vi "Report - Flow Control.vi"(0 "Log Folder Path (Create Log)":path, 1 "DUT Number":i32, 2 "Text Input":string[](array[string]), 3 "WLAN TX Result":T8, 4 "WLAN RX Result":T7, 5 "error in":errorcluster, 6 "Reprot Log Flow Control":T6, 7 "DUT log path":path, 8 "TV Parameters(DataType)":T1 {"Standard" items=["80211A/G/J/P OFDM", "80211B/G DSSS", "80211G DSSSOFDM", "80211N MIMOOFDM", "80211AC MIMOOFDM"]; "OFDM Data Rate (Mbps)" items=["6", "9", "12", "18", "24", "36", "48", "54"]; "80211n PLCP Frame Format" items=["Mixed Format", "Greenfield Format"]; "FEC Coding Type" items=["BCC", "LDPC"]; "DSSS Data Rate (Mbps)" items=["1", "2", "5.5 CCK", "5.5 PBCC", "11 CCK", "11 PBCC", "22", "33"]}) -> (14 "Pass or not":bool, 15 "Text Output":string[](array[string]), 16 "Cluster 2":T2, 17 "DUT1 log path":path, 19 "error out":errorcluster)   [LabVIEW 2014]
uses:
  TypeDef/Report Log Flow Control.ctl
  TV/RW/Includes/WLAN - TV - RW - INC - TV_DataType_Cluster.ctl
  TypeDef/DUT Number.ctl
  <vilib>/Utility/file.llb/Write To Spreadsheet File (string).vi
  <vilib>/Utility/file.llb/Read From Spreadsheet File (string).vi
panel:
  out "DUT1 Results":string[][](array[string])
  out "Text Output":string[][](array[string])
  in  "BT RX Result":T3
  in  "BT TX EDR Result":T4 {"EDR_OMEGA_I (Hz)" format="%.2g"; "EDR_PROB_EVM_99_PASS (%)" format="%.2g"; "EDR_EVM_PK (%)" format="%.2g"; "EDR_EVM_AV (%)" format="%.2g"; "EDR_POW_DIFF_DB (dB)" format="%.2f"; "POWER_PEAK_DBM (dBm)" format="%.2f"; "POWER_AVERAGE_DBM (dBm)" format="%.2f"}
  in  "BT TX BR Result":T5 {"FREQ_EST_HEADER  (Hz)" format="%^.3g"; "FREQ_EST (Hz)" format="%^.3e"; "FREQ_DRIFT (Hz)" format="%^.3e"; "DELTA_F2_MAX_ACCESS (Hz)" format="%^.3e"; "DELTA_F2_AVERAGE (Hz)" format="%^.3e"; "POWER_PEAK_DBM (dBm)" format="%.2f"; "POWER_AVERAGE_DBM (dBm)" format="%.2f"; "DELTA_F1_AVERAGE (Hz)" format="%^.3e"}
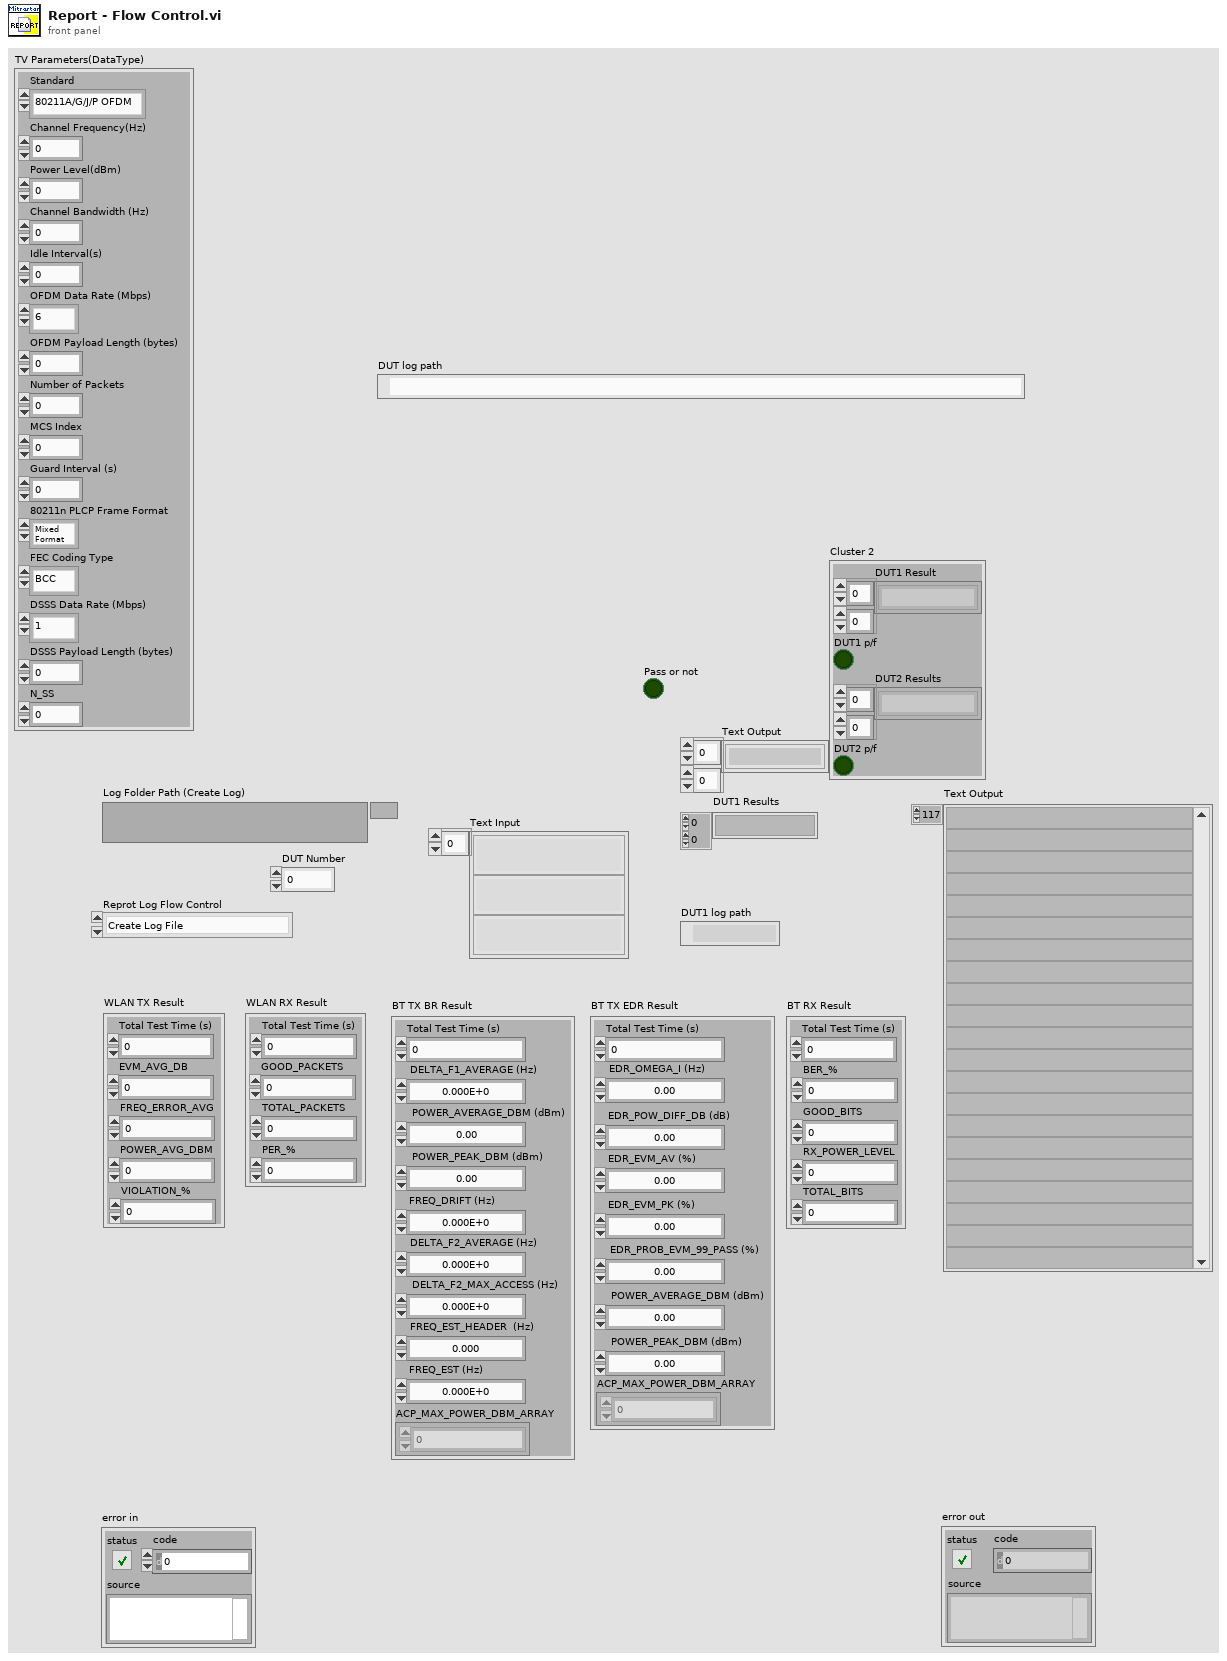
[diagram p1: front panel]
types:
  T1 = typedef "WLAN - TV - RW - INC - TV_DataType_Cluster.ctl" = cluster{"Standard":i32, "Channel Frequency(Hz)":dbl, "Power Level(dBm)":dbl, "Channel Bandwidth (Hz)":dbl, "Idle Interval(s)":dbl, "OFDM Data Rate (Mbps)":i32, "OFDM Payload Length (bytes)":i32, "Number of Packets":i32, "MCS Index":i32, "Guard Interval (s)":dbl, "80211n PLCP Frame Format":i32, "FEC Coding Type":i32, "DSSS Data Rate (Mbps)":i32, "DSSS Payload Length (bytes)":i32, "N_SS":i32}
  T2 = cluster{"DUT1 Result":string[][], "DUT1 p/f":bool, "DUT2 Results":string[][], "DUT2 p/f":bool}
  T3 = cluster{"Total Test Time (s)":dbl, "BER_%":dbl, "GOOD_BITS":i32, "RX_POWER_LEVEL":dbl, "TOTAL_BITS":i32}
  T4 = cluster{"Total Test Time (s)":dbl, "EDR_OMEGA_I (Hz)":dbl, "EDR_POW_DIFF_DB (dB)":dbl, "EDR_EVM_AV (%)":dbl, "EDR_EVM_PK (%)":dbl, "EDR_PROB_EVM_99_PASS (%)":dbl, "POWER_AVERAGE_DBM (dBm)":dbl, "POWER_PEAK_DBM (dBm)":dbl, "ACP_MAX_POWER_DBM_ARRAY":dbl[]}
  T5 = cluster{"Total Test Time (s)":dbl, "DELTA_F1_AVERAGE (Hz)":dbl, "POWER_AVERAGE_DBM (dBm)":dbl, "POWER_PEAK_DBM (dBm)":dbl, "FREQ_DRIFT (Hz)":dbl, "DELTA_F2_AVERAGE (Hz)":dbl, "DELTA_F2_MAX_ACCESS (Hz)":dbl, "FREQ_EST_HEADER  (Hz)":dbl, "FREQ_EST (Hz)":dbl, "ACP_MAX_POWER_DBM_ARRAY":dbl[]}
  T6 = typedef "Report Log Flow Control.ctl" = enum16{"Create Log File", "Append Test Item Head", "Append WLAN TX IQ Result", "Append WLAN TX Spectrum Result", "Append WLAN RX Result", "Append BT TX BR Result", "Append BT TX EDR Result", "Append Customized Text", "Append BT RX Result", "Read Log File", "Save Test Time"}
  T7 = cluster{"Total Test Time (s)":dbl, "GOOD_PACKETS":i32, "TOTAL_PACKETS":i32, "PER_%":dbl}
  T8 = cluster{"Total Test Time (s)":dbl, "EVM_AVG_DB":dbl, "FREQ_ERROR_AVG":dbl, "POWER_AVG_DBM":dbl, "VIOLATION_%":dbl}
  T9 = typedef "DUT Number.ctl" = string
  T10 = cluster{"all rows":string[][], "p/f":bool, "all rows":string[][], "p/f":bool}
  T11 = cluster{"POWER_AVG_DBM":string, "EVM_AVG_DB":string, "FREQ_ERROR_AVG":string, "RX_PER":string}
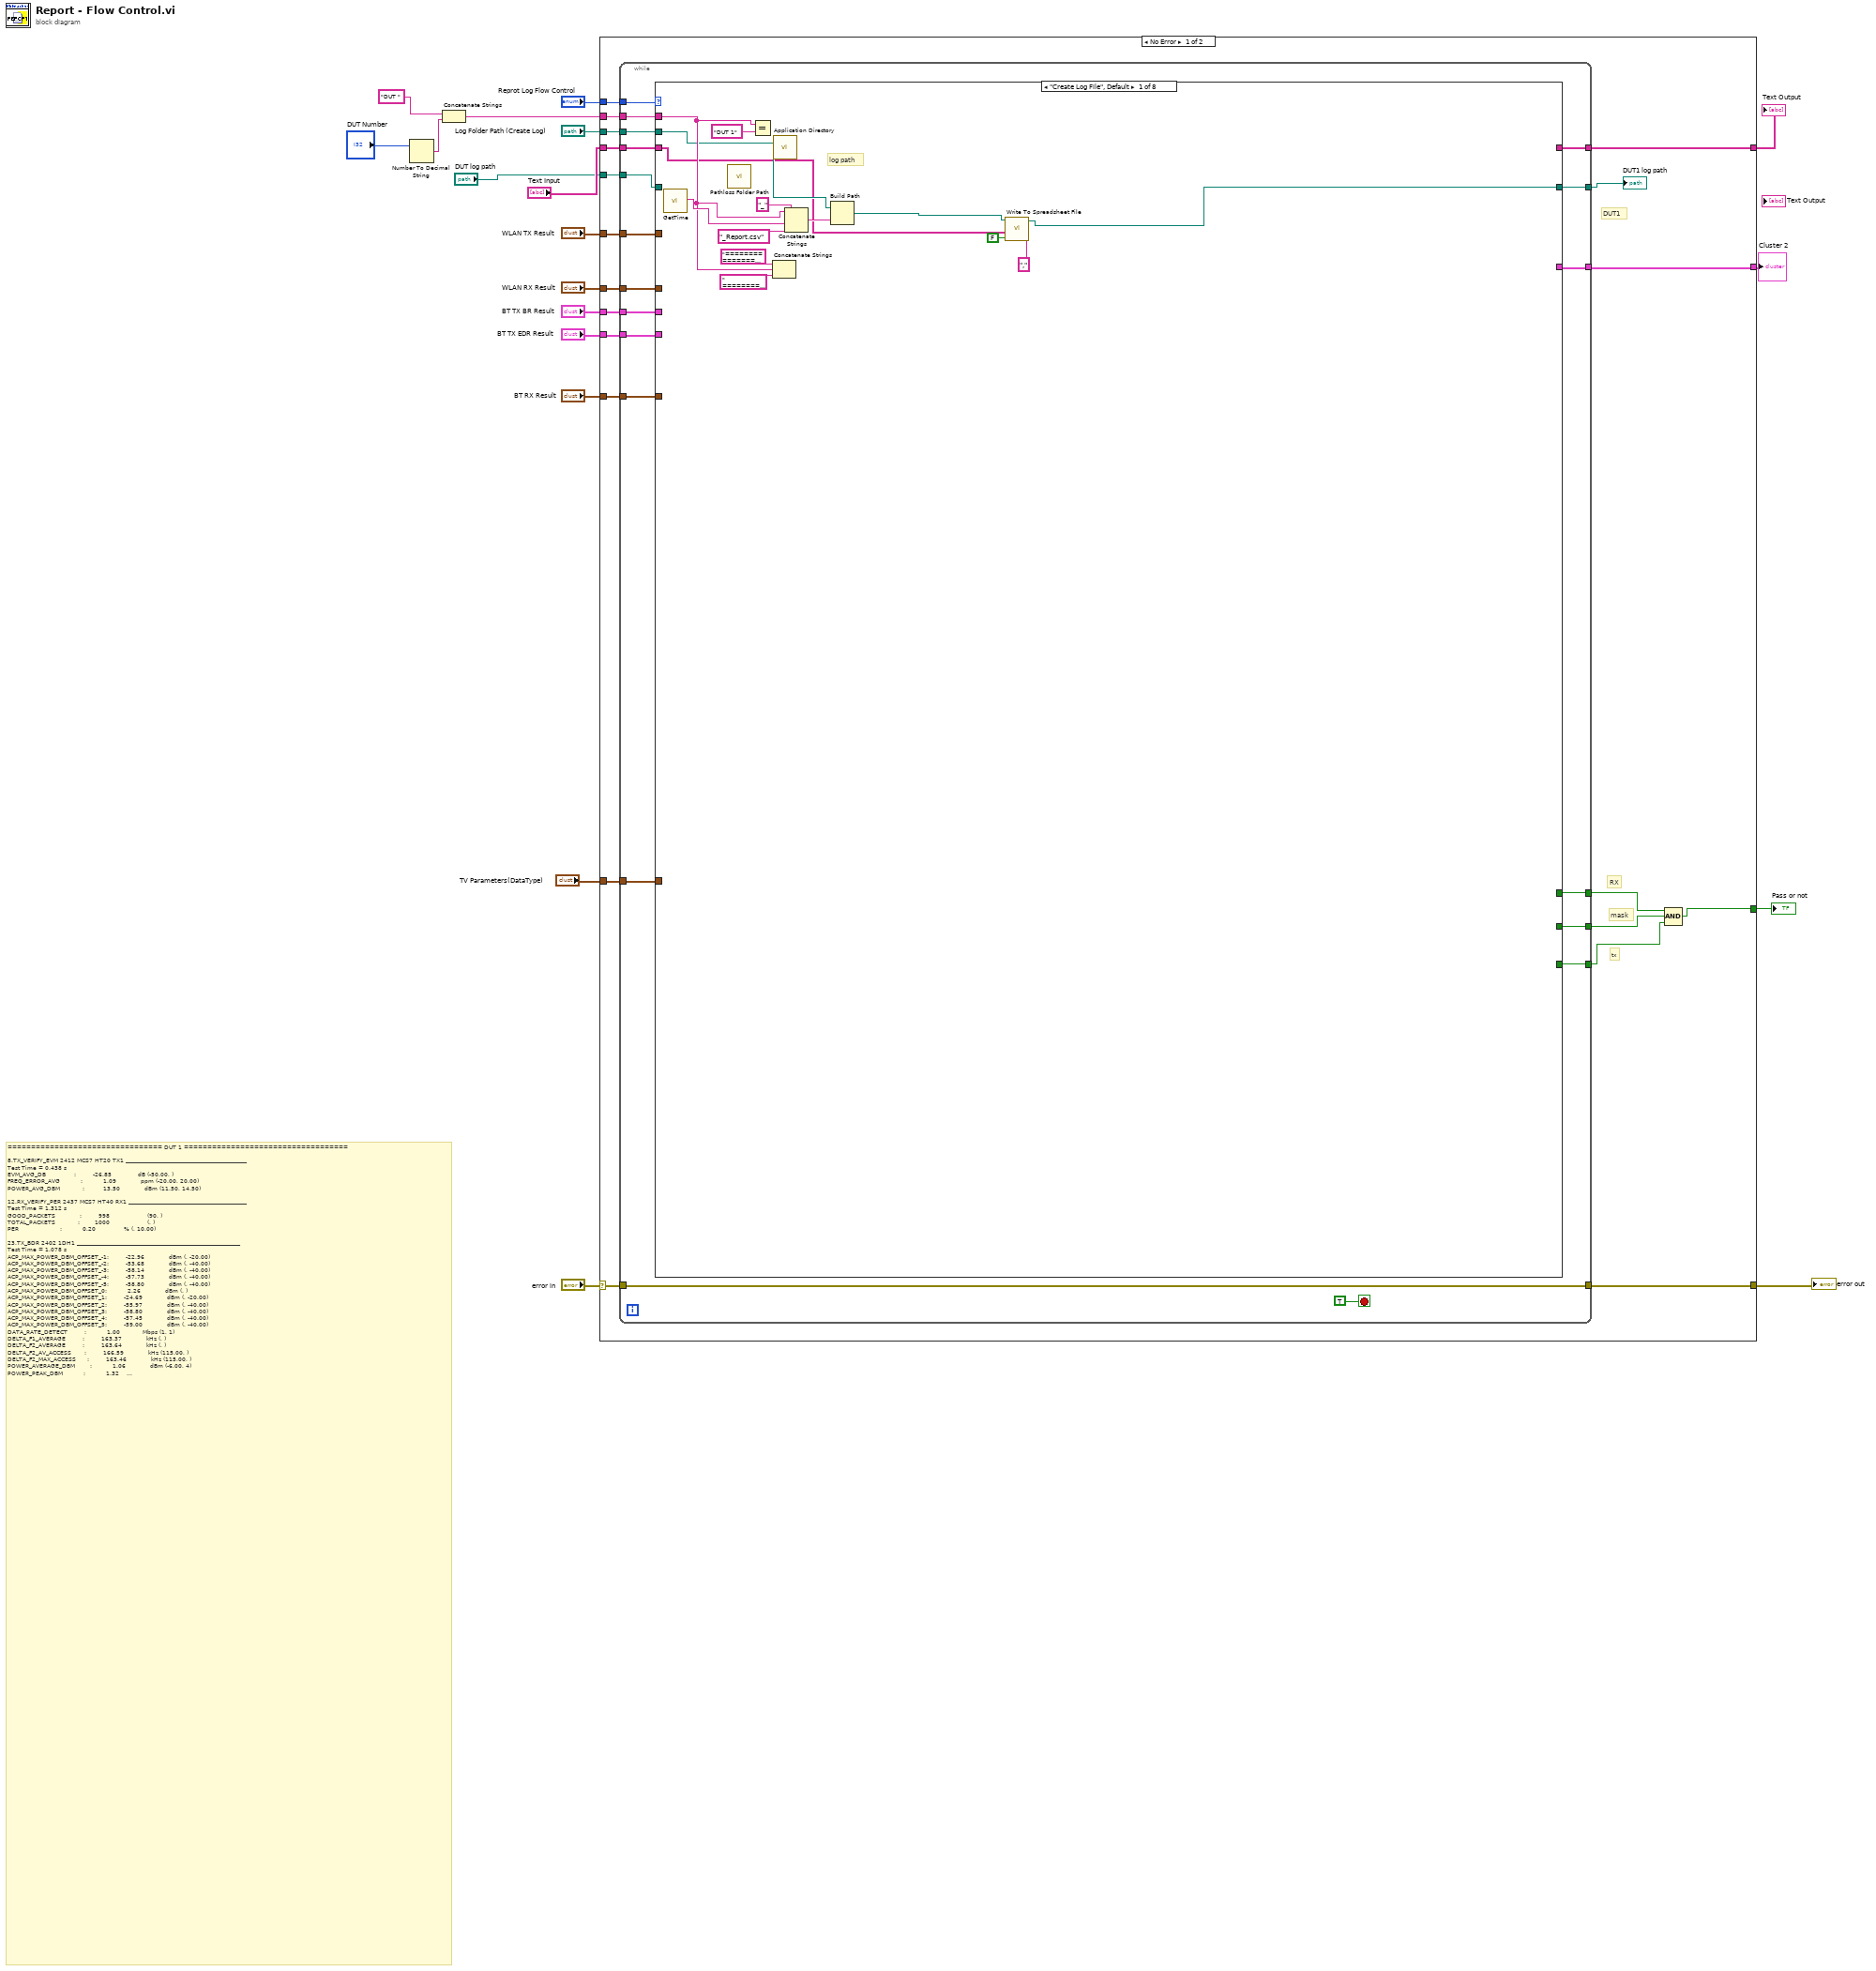
[diagram p0: block diagram]
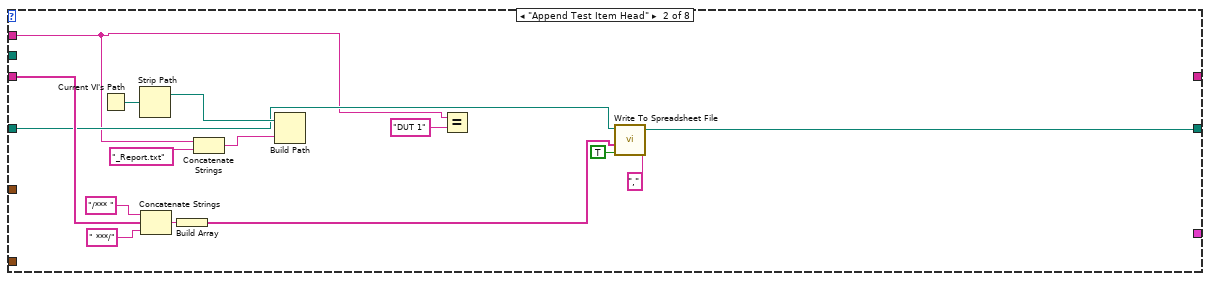
[diagram p2: hidden frame]
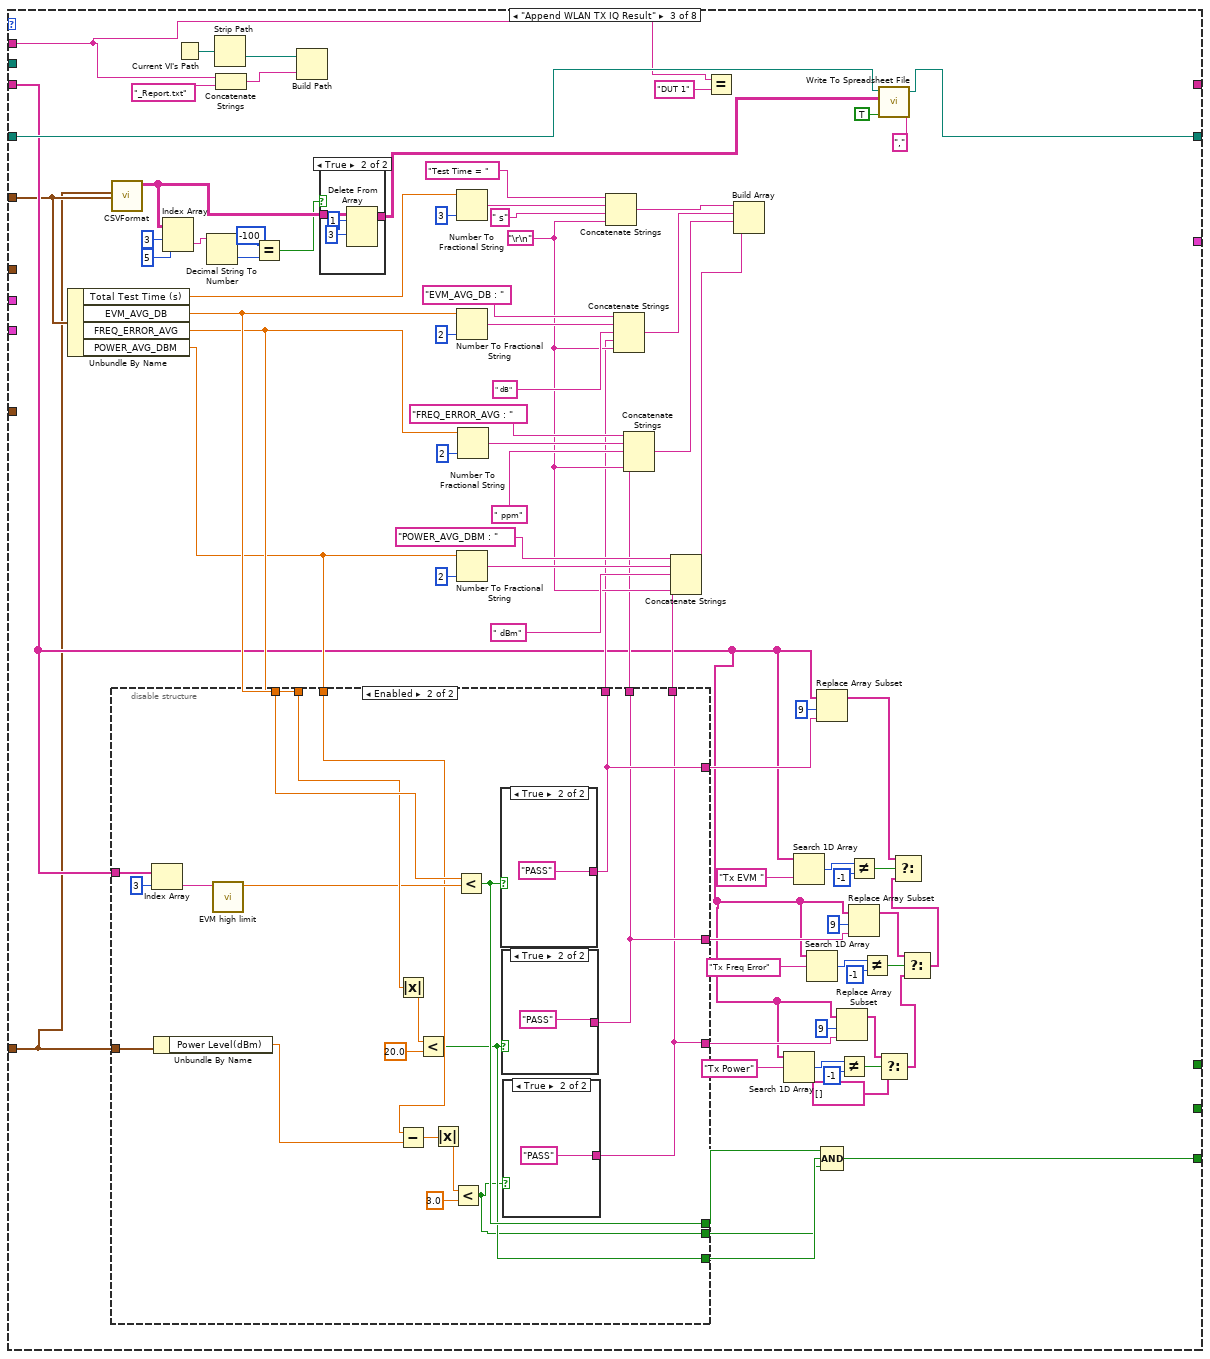
[diagram p3: hidden frame]
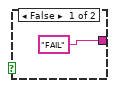
[diagram p6: hidden frame]
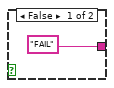
[diagram p7: hidden frame]
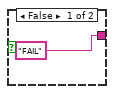
[diagram p8: hidden frame]
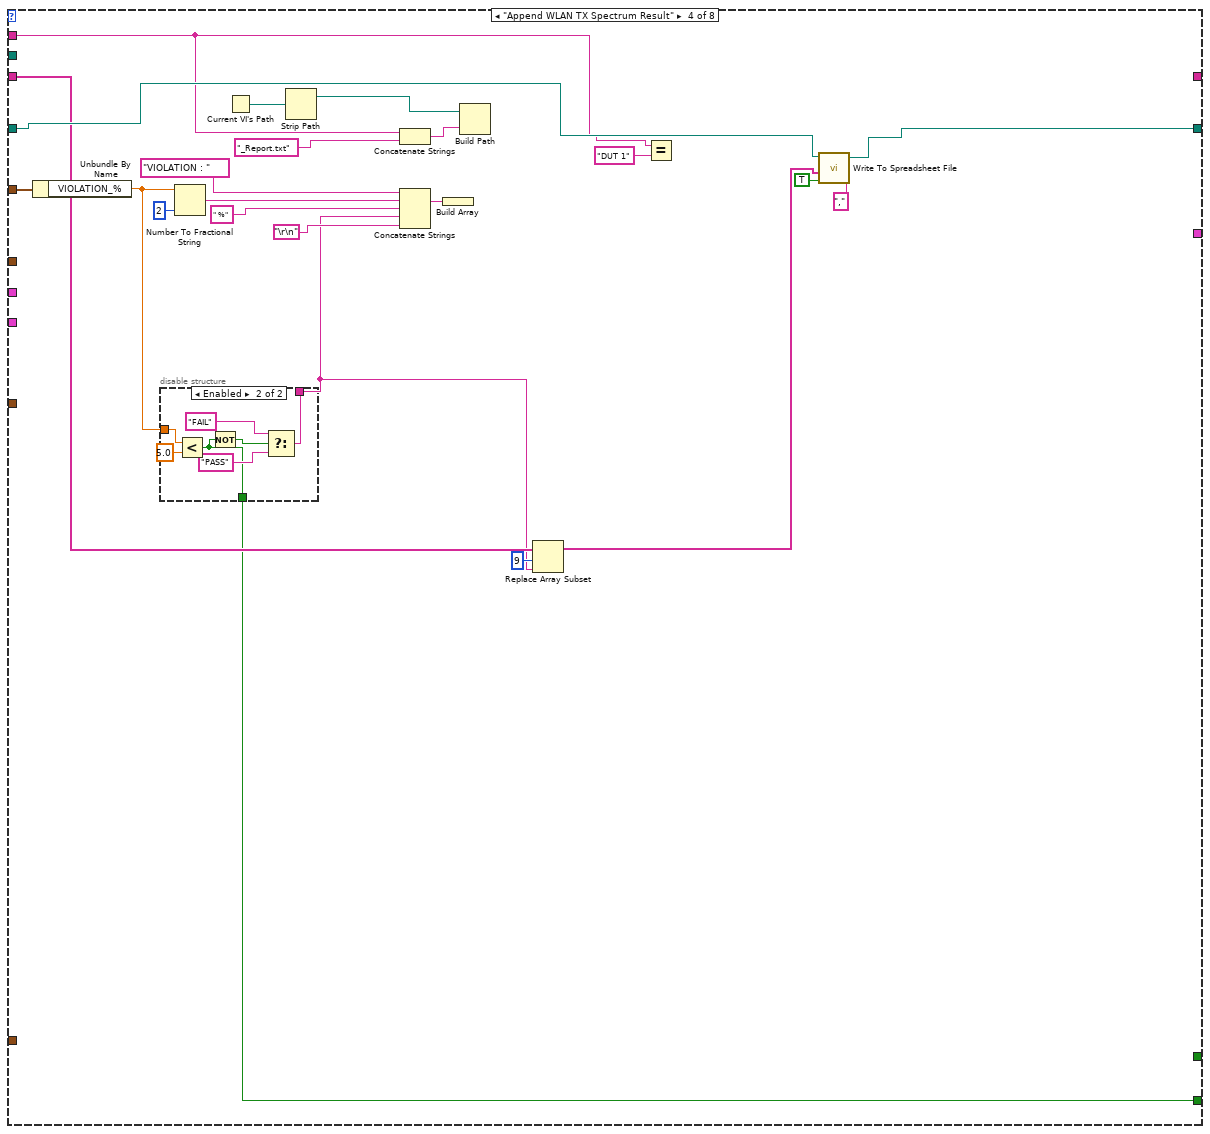
[diagram p9: hidden frame]
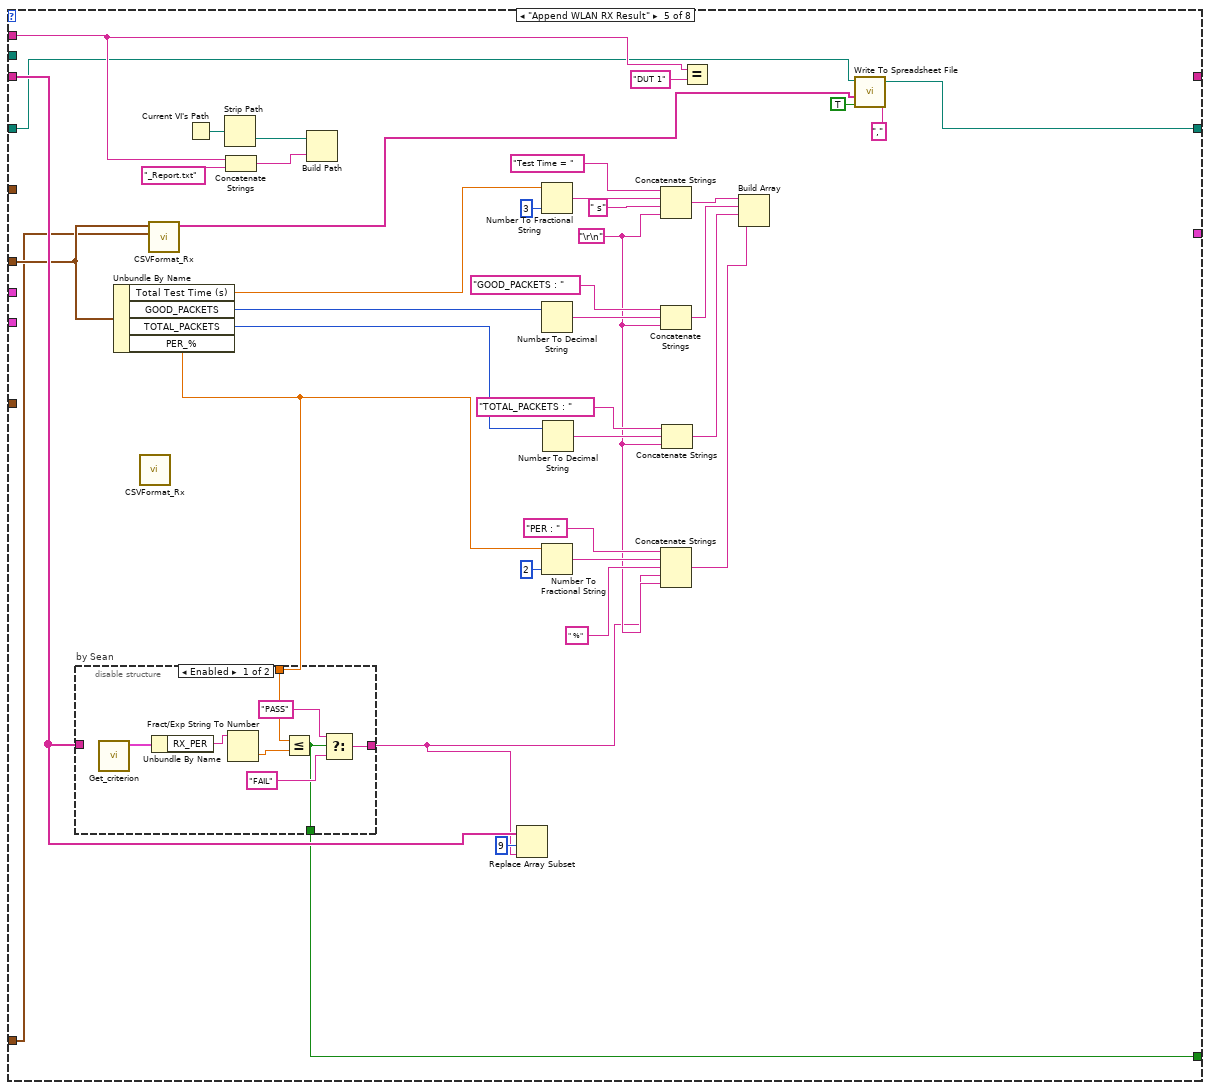
[diagram p11: hidden frame]
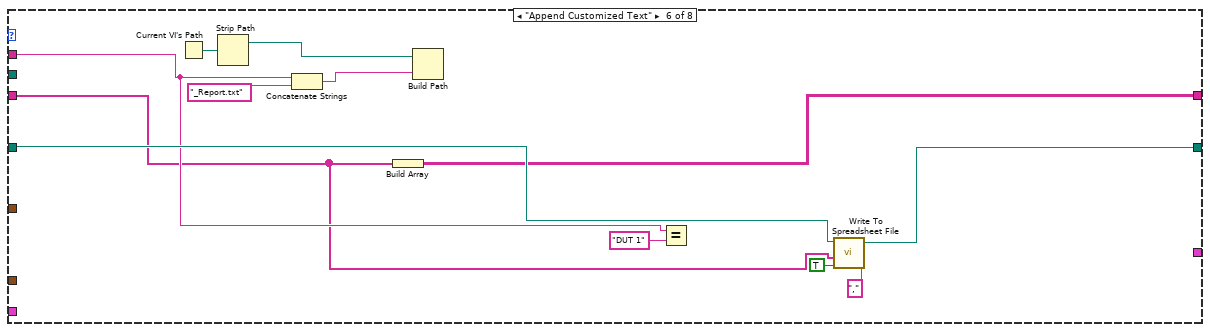
[diagram p13: hidden frame]
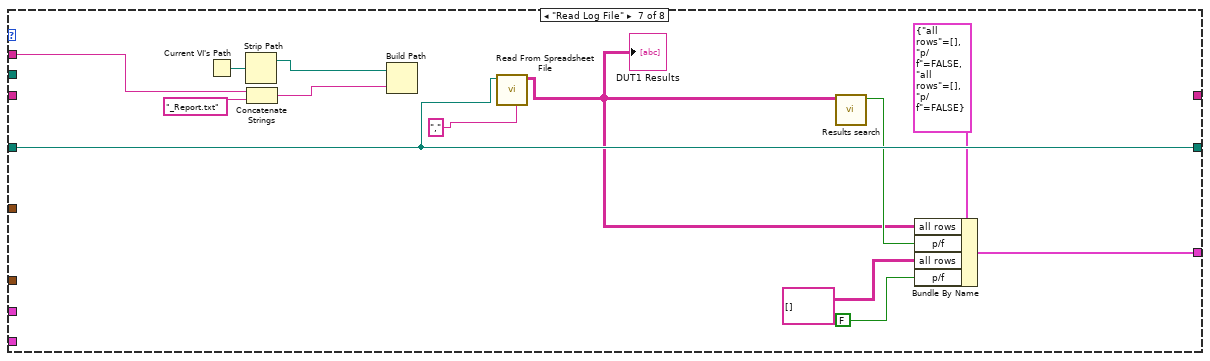
[diagram p14: hidden frame]
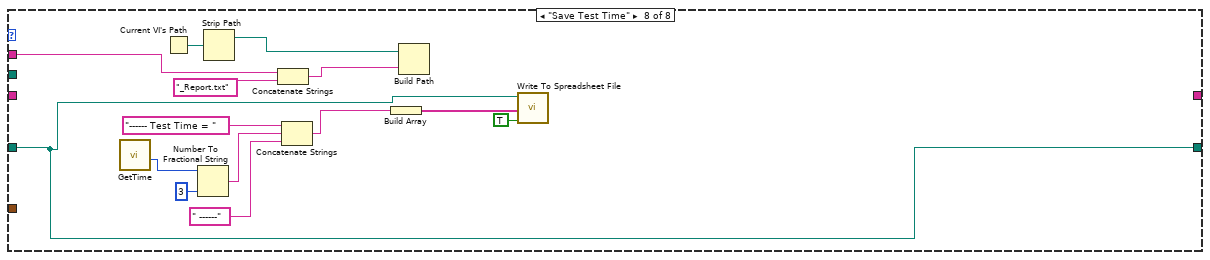
[diagram p15: hidden frame]
diagram:
  # "================================= DUT 1 ===================================\n\n8.TX_VERIFY_EVM 2412 MCS7 HT20 TX1 ___________________________________________\nTest Time = 0.438 s\nEVM_AVG_DB               :         -26.85              dB (-50.00, )\nFREQ_ERROR_AVG           :           1.09             ppm (-20.00, 20.00)\nPOWER_AVG_DBM            :          13.50             dBm (11.50, 14.50)\n\n12.RX_VERIFY_PER 2437 MCS7 HT40 RX1 __________________________________________\nTest Time = 1.312 s\nGOOD_PACKETS             :         998                    (90, )\nTOTAL_PACKETS            :        1000                    (, )\nPER                      :           0.20               % (, 10.00)\n\n23.TX_BDR 2402 1DH1 __________________________________________________________\nTest Time = 1.078 s\nACP_MAX_POWER_DBM_OFFSET_-1:         -22.96             dBm (, -20.00)\nACP_MAX_POWER_DBM_OFFSET_-2:         -53.68             dBm (, -40.00)\nACP_MAX_POWER_DBM_OFFSET_-3:         -58.14             dBm (, -40.00)\nACP_MAX_POWER_DBM_OFFSET_-4:         -57.73             dBm (, -40.00)\nACP_MAX_POWER_DBM_OFFSET_-5:         -58.80             dBm (, -40.00)\nACP_MAX_POWER_DBM_OFFSET_0:           2.26             dBm (, )\nACP_MAX_POWER_DBM_OFFSET_1:         -24.69             dBm (, -20.00)\nACP_MAX_POWER_DBM_OFFSET_2:         -55.97             dBm (, -40.00)\nACP_MAX_POWER_DBM_OFFSET_3:         -58.80             dBm (, -40.00)\nACP_MAX_POWER_DBM_OFFSET_4:         -57.45             dBm (, -40.00)\nACP_MAX_POWER_DBM_OFFSET_5:         -59.00             dBm (, -40.00)\nDATA_RATE_DETECT         :           1.00            Mbps (1, 1)\nDELTA_F1_AVERAGE         :         163.37             kHz (, )\nDELTA_F2_AVERAGE         :         163.64             kHz (, )\nDELTA_F2_AV_ACCESS       :         166.59             kHz (115.00, )\nDELTA_F2_MAX_ACCESS      :         163.46             kHz (115.00, )\nPOWER_AVERAGE_DBM        :           1.06             dBm (-6.00, 4)\nPOWER_PEAK_DBM           :           1.32             dBm (, 23.00)\n\n24.TX_EDR 2402 2DH1 __________________________________________________________\nTest Time = 0.344 s\nACP_MAX_POWER_DBM_OFFSET_-2:         -41.51             dBm (, -20.00)\nACP_MAX_POWER_DBM_OFFSET_-3:         -51.70             dBm (, -40.00)\nACP_MAX_POWER_DBM_OFFSET_-4:         -52.15             dBm (, -40.00)\nACP_MAX_POWER_DBM_OFFSET_-5:         -53.92             dBm (, -40.00)\nACP_MAX_POWER_DBM_OFFSET_0:          -1.67             dBm (, )\nACP_MAX_POWER_DBM_OFFSET_2:         -43.45             dBm (, -20.00)\nACP_MAX_POWER_DBM_OFFSET_3:         -51.34             dBm (, -40.00)\nACP_MAX_POWER_DBM_OFFSET_4:         -51.38             dBm (, -40.00)\nACP_MAX_POWER_DBM_OFFSET_5:         -53.06             dBm (, -40.00)\nACP_MAX_POWER_DB_OFFSET_-1:         -40.81              dB (, -26.00)\nACP_MAX_POWER_DB_OFFSET_1:         -42.10              dB (, -26.00)\nEDR_EVM_AV               :           0.03                 (, 13.00)\nEDR_EVM_PK               :           0.07                 (, 25.00)\nEDR_EXTREME_OMEGA_0      :           3.75             kHz (-10.00, 10.00)\nEDR_EXTREME_OMEGA_I0     :         -14.61             kHz (-75.00, 75.00)\nEDR_OMEGA_I              :         -18.12             kHz (-75.00, 75.00)\nEDR_POW_DIFF_DB          :           0.29              dB (-4.00, 1)\nEDR_PROB_EVM_99_PASS     :         100.00               % (100.00, 100.00)\nPOWER_AVERAGE_DBM        :           1.20             dBm (-6.00, 4)\nPOWER_PEAK_DBM           :           4.10             dBm (, 23.00)\n\n26.RX_BDR 2402 1DH1 __________________________________________________________\nTest Time = 4.203 s\nBER                      :           0.00               % (, 0.10)\nGOOD_BITS                :       30240.00            bits (, ))\nRX_POWER_LEVEL           :         -70.00             dBm (, )\nTOTAL_BITS               :       30240.00            bits (, )\n\n      \n27.RX_EDR 2441 2DH1 __________________________________________________________\nTest Time = 0.422 s\nBER                      :           0.00               % (, 0.10)\nGOOD_BITS                :       30672.00            bits (, )\nRX_POWER_LEVEL           :         -70.00             dBm (, )\nTOTAL_BITS               :       30672.00            bits (, )"
  n1 = Number To Decimal String(number="DUT Number") -> (decimal integer string=w3:string)  [unwired: 1 in]
  n2 = Concatenate Strings("DUT ", w3) -> (w2:string)
  n3 = case shown="No Error" "error in" {
    selector: "error in" -> [w30 w311]
    tunnel: "Reprot Log Flow Control" -> [w39 _]
    tunnel: w2 -> [w38 _]
    tunnel: "Log Folder Path (Create Log)" -> [w37 _]
    tunnel: "Text Input" -> [w36 _]
    tunnel: "WLAN TX Result" -> [w35 _]
    tunnel: "WLAN RX Result" -> [w34 _]
    tunnel: "BT TX BR Result" -> [w33 _]
    tunnel: "BT TX EDR Result" -> [w32 _]
    tunnel: "BT RX Result" -> [w31 _]
    tunnel: [w29 w311] -> w11
    tunnel: [w28 _] -> w9
    tunnel: [w27 _] -> w8
    tunnel: [w23 _] -> w7
    tunnel: "TV Parameters(DataType)" -> [w22 _]
    tunnel: "DUT log path" -> [w21 _]
    frame No Error {
      # "tx"
      # "mask"
      # "RX"
      # "DUT1"
      n4 = while {
        tunnel: w39 -> [w57]
        tunnel: w38 -> [w56]
        tunnel: w37 -> [w42]
        tunnel: w36 -> [w55]
        tunnel: w35 -> [w54]
        tunnel: w34 -> [w53]
        tunnel: w33 -> [w52]
        tunnel: w32 -> [w51]
        tunnel: w31 -> [w50]
        tunnel: [w49] -> w29
        tunnel: w30 -> [w49]
        tunnel: [w48] -> w28
        tunnel: [w47] -> w27
        tunnel: [w46] -> w24
        tunnel: [w45] -> w25
        tunnel: [w44] -> w26
        tunnel: w22 -> [w43]
        tunnel: [w41] -> w20
        tunnel: w21 -> [w40]
        stop <- TRUE stop-if-true
        n5 = case shown="\"Create Log File\", Default" w57 {
          tunnel: w56 -> [w67 w76 w130 w204 w236 w276 w292 w302]
          tunnel: w42 -> [w64 _ _ _ _ _ _ _]
          tunnel: [w60 w73 w129 w203 w237 w277 w291 w298] -> w41
          tunnel: w40 -> [_ w78 w131 w205 w231 w278 w291 w298]
          tunnel: w55 -> [w62 w80 w104 w202 w235 w272 _ _]
          tunnel: w54 -> [_ _ w97 w218 _ _ _ _]
          tunnel: w53 -> [_ _ _ _ w228 _ _ _]
          tunnel: w52 -> [_ _ _ _ _ _ _ _]
          tunnel: w51 -> [_ _ _ _ _ _ _ _]
          tunnel: w50 -> [_ _ _ _ _ _ _ _]
          tunnel: [_ _ _ _ _ w273 _ _] -> w48
          tunnel: [_ _ _ _ _ _ w287 _] -> w47
          tunnel: [_ _ w100 _ _ _ _ _] -> w46
          tunnel: [_ _ _ w198 _ _ _ _] -> w45
          tunnel: [_ _ _ _ w232 _ _ _] -> w44
          tunnel: w43 -> [_ _ w96 _ w227 _ _ _]
          frame "Create Log File", Default {
            # "log path"
            n6 = call "GetTime.vi"() -> ("TimeStringForPath"=w70:string)  [unwired: 8 in, 3 out]
            n7 = call "Pathloss Folder Path.vi"() -> ()  [unwired: 11 in, 1 out]
            n8 = Equal?(x=w67, y=T9 "DUT 1") -> ()  [unwired: 1 out]
            n9 = Concatenate Strings("================================= ", w67, " ===================================") -> ()  [unwired: 1 out]
            n10 = call <vilib>:"Application Directory.vi"() -> ()  [unwired: 1 out]
            n11 = Concatenate Strings(w67, T9 "_" ("string"), w70, "_Report.csv" ("string")) -> (w65:string)
            n12 = Build Path(base path=w64, name or relative path=w65) -> (appended path=w63:path)
            n13 = call-poly <vilib>:"Write To Spreadsheet File.vi"("delimiter (\\t)"="," ("delimiter (\\t)"), "append to file? (new file:F)"=FALSE, "1D data"=w62, "file path (dialog if empty)"=w63) -> ("new file path (Not A Path if cancelled)"=w60:path)  [unwired: 4 in]
          }
          frame "Append Test Item Head" {
            n14 = Current VI's Path() -> (path=w82:path)
            n15 = Strip Path(path=w82) -> (stripped path=w81:path)  [unwired: 1 out]
            n16 = Concatenate Strings("/*** " ("string"), w80, " ***/" ("string")) -> (w87:string)
            n17 = Build Array(w87) -> (w79:string[])
            n18 = Concatenate Strings(w76, "_Report.txt" ("string")) -> (w83:string)
            n19 = Build Path(base path=w81, name or relative path=w83) -> ()  [unwired: 1 out]
            n20 = Equal?(x=w76, y=T9 "DUT 1") -> ()  [unwired: 1 out]
            n21 = call-poly <vilib>:"Write To Spreadsheet File.vi"("delimiter (\\t)"="," ("delimiter (\\t)"), "append to file? (new file:F)"=TRUE, "1D data"=w79, "file path (dialog if empty)"=w78) -> ("new file path (Not A Path if cancelled)"=w73:path)  [unwired: 4 in]
          }
          frame "Append WLAN TX IQ Result" {
            w136 = "\r\n"
            n22 = Unbundle By Name(w97) -> ("Total Test Time (s)"=w140:dbl, "EVM_AVG_DB"=w139:dbl, "FREQ_ERROR_AVG"=w138:dbl, "POWER_AVG_DBM"=w137:dbl)
            n23 = call "CSVFormat.vi"("TV Parameters(DataType)"=w96, "WLAN TX Result"=w97) -> ("Array"=w94:string[][])  [unwired: 9 in]
            n24 = disable-structure shown="Enabled" {
              disable-tunnel: w104 -> [_ w182]
              disable-tunnel: w139 -> [_ w189]
              disable-tunnel: w138 -> [_ w188]
              disable-tunnel: w137 -> [_ w176]
              disable-tunnel: [_ w186] -> w135
              disable-tunnel: [_ w185] -> w134
              disable-tunnel: [_ w184] -> w133
              disable-tunnel: [_ w186] -> w127
              disable-tunnel: [_ w185] -> w116
              disable-tunnel: [_ w184] -> w108
              disable-tunnel: [_ w174] -> w103
              disable-tunnel: [_ w173] -> w102
              disable-tunnel: [_ w172] -> w101
              disable-tunnel: w96 -> [_ w171]
              frame Disabled {
              }
              frame Enabled {
                n25 = Index Array(array=w182, index=3) -> (element=w180:string)
                n26 = Unbundle By Name(w171) -> ("Power Level(dBm)"=w170:dbl)
                n27 = call "EVM high limit.vi"("MCS Index"=w180) -> ("EVM High Limit"=w183:dbl)  [unwired: 10 in]
                n28 = Absolute Value(x=w188) -> (abs(x)=w187:dbl)
                n29 = Subtract(x=w176, y=w170) -> (x-y=w175:dbl)
                n30 = Less?(x=w187, y=20.0) -> (x < y?=w173:bool)
                n31 = Absolute Value(x=w175) -> (abs(x)=w179:dbl)
                n32 = Less?(x=w179, y=3.0 ("upper limit")) -> (x < y?=w172:bool)
                n33 = Less?(x=w189, y=w183) -> (x < y?=w174:bool)
                n34 = case shown="True" w174 {
                  tunnel: ["FAIL" ("string") "PASS" ("string")] -> w186
                  frame False {
                  }
                  frame True {
                  }
                }
                n35 = case shown="True" w173 {
                  tunnel: ["FAIL" ("string") "PASS" ("string")] -> w185
                  frame False {
                  }
                  frame True {
                  }
                }
                n36 = case shown="True" w172 {
                  tunnel: ["FAIL" ("string") "PASS" ("string")] -> w184
                  frame False {
                  }
                  frame True {
                  }
                }
              }
            }
            n37 = Index Array(array=w94, index (row)=3, index (col)=5 ("disabled index (col)")) -> (element=w91:string)
            n38 = Current VI's Path() -> (path=w142:path)
            n39 = Decimal String To Number(string=w91) -> (number=w90:i32)  [unwired: 2 in, 1 out]
            n40 = Strip Path(path=w142) -> (stripped path=w141:path)  [unwired: 1 out]
            n41 = Concatenate Strings(w130, "_Report.txt" ("string")) -> (w143:string)
            n42 = Equal?(x=-100, y=w90) -> (x = y?=w88:bool)
            n43 = Build Path(base path=w141, name or relative path=w143) -> ()  [unwired: 1 out]
            n44 = case shown="True" w88 {
              tunnel: w94 -> [w165 w169]
              tunnel: [w165 w166] -> w95
              frame False {
              }
              frame True {
                n45 = Delete From Array(array=w169, length=1, index (row)=3) -> (array with subset deleted=w166:string[][])  [unwired: 1 in, 1 out]
              }
            }
            n46 = Number To Fractional String(number=w140, precision (6)=i16 3) -> (F-format string=w162:string)  [unwired: 2 in]
            n47 = Number To Fractional String(number=w139, precision (6)=i16 2) -> (F-format string=w157:string)  [unwired: 2 in]
            n48 = Number To Fractional String(number=w137, precision (6)=i16 2) -> (F-format string=w148:string)  [unwired: 2 in]
            n49 = Number To Fractional String(number=w138, precision (6)=i16 2) -> (F-format string=w155:string)  [unwired: 2 in]
            n50 = Concatenate Strings("Test Time = ", w162, " s" ("string"), w136) -> (w160:string)
            n51 = Concatenate Strings("EVM_AVG_DB : " ("string"), w157, " dB" ("string"), w135, w136) -> (w147:string)
            n52 = Concatenate Strings("FREQ_ERROR_AVG : " ("string"), w155, " ppm" ("string"), w134, w136) -> (w146:string)
            n53 = Concatenate Strings("POWER_AVG_DBM : " ("string"), w148, " dBm" ("string"), w133, w136) -> (w145:string)
            n54 = Equal?(x=w130, y=T9 "DUT 1") -> ()  [unwired: 1 out]
            n55 = Build Array(w160, w147, w146, w145) -> ()  [unwired: 1 out]
            n56 = Search 1D Array(1D array=w104, element="Tx Power" ("new element/subarray")) -> (index of element=w111:i32)  [unwired: 1 in]
            n57 = Search 1D Array(1D array=w104, element="Tx EVM ") -> (index of element=w125:i32)  [unwired: 1 in]
            n58 = Search 1D Array(1D array=w104, element="Tx Freq Error" ("new element/subarray")) -> (index of element=w120:i32)  [unwired: 1 in]
            n59 = Replace Array Subset(array=w104, new element=w127, index=9) -> (w122:string[])
            n60 = Compound Arithmetic op=AND(w103, w102, w101) -> (w100:bool)
            n61 = Replace Array Subset(array=w104, new element=w108, index=9) -> (w107:string[])
            n62 = Not Equal?(x=w111, y=-1) -> (x != y?=w113:bool)
            n63 = Not Equal?(x=w125, y=-1) -> (x != y?=w123:bool)
            n64 = Replace Array Subset(array=w104, new element=w116, index=9) -> (w115:string[])
            n65 = Not Equal?(x=w120, y=-1) -> (x != y?=w118:bool)
            n66 = call-poly <vilib>:"Write To Spreadsheet File.vi"("delimiter (\\t)"="," ("delimiter (\\t)"), "append to file? (new file:F)"=TRUE, "2D data"=w95, "file path (dialog if empty)"=w131) -> ("new file path (Not A Path if cancelled)"=w129:path)  [unwired: 4 in]
            n67 = Select(t=w107, s=w113, f=string[] []) -> (s? t:f=w106:string[])
            n68 = Select(t=w115, s=w118, f=w106) -> (s? t:f=w114:string[])
            n69 = Select(t=w122, s=w123, f=w114) -> ()  [unwired: 1 out]
          }
          frame "Append WLAN TX Spectrum Result" {
            n70 = Unbundle By Name(w218) -> ("VIOLATION_%"=w208:dbl)
            n71 = disable-structure shown="Enabled" {
              disable-tunnel: w208 -> [_ w222]
              disable-tunnel: [_ w223] -> w200
              disable-tunnel: [_ w219] -> w198
              frame Disabled {
              }
              frame Enabled {
                n72 = Less?(x=w222, y=5.0) -> (x < y?=w219:bool)
                n73 = Not(x=w219) -> (.not. x?=w220:bool)
                n74 = Select(t="FAIL", s=w220, f="PASS") -> (s? t:f=w223:string)
              }
            }
            n75 = Number To Fractional String(number=w208, precision (6)=i16 2) -> (F-format string=w215:string)  [unwired: 2 in]
            n76 = Current VI's Path() -> (path=w210:path)
            n77 = Strip Path(path=w210) -> (stripped path=w209:path)  [unwired: 1 out]
            n78 = Concatenate Strings(w204, "_Report.txt" ("string")) -> (w211:string)
            n79 = Concatenate Strings("VIOLATION : " ("string"), w215, " %" ("string"), w200, "\r\n") -> (w213:string)
            n80 = Build Array(w213) -> ()  [unwired: 1 out]
            n81 = Build Path(base path=w209, name or relative path=w211) -> ()  [unwired: 1 out]
            n82 = Replace Array Subset(array=w202, new element=w200, index=9) -> (w199:string[])
            n83 = Equal?(x=w204, y=T9 "DUT 1") -> ()  [unwired: 1 out]
            n84 = call-poly <vilib>:"Write To Spreadsheet File.vi"("delimiter (\\t)"="," ("delimiter (\\t)"), "append to file? (new file:F)"=TRUE, "1D data"=w199, "file path (dialog if empty)"=w205) -> ("new file path (Not A Path if cancelled)"=w203:path)  [unwired: 4 in]
          }
          frame "Append WLAN RX Result" {
            w239 = "\r\n"
            n85 = Unbundle By Name(w228) -> ("Total Test Time (s)"=w241:dbl, "GOOD_PACKETS"=w256:i32, "TOTAL_PACKETS"=w253:i32, "PER_%"=w240:dbl)
            n86 = disable-structure "by Sean" shown="Enabled" {
              disable-tunnel: w235 -> [_ _]
              disable-tunnel: w240 -> [w269 _]
              disable-tunnel: [w265 _] -> w233
              disable-tunnel: [w264 _] -> w232
              frame Enabled {
                n87 = call "Get_criterion.vi"() -> ("WLAN_Range"=w271:T11)  [unwired: 9 in, 2 out]
                n88 = Unbundle By Name(w271) -> ("RX_PER"=w270:string)
                n89 = Fract/Exp String To Number(string=w270) -> (number=w268:dbl)  [unwired: 3 in, 1 out]
                n90 = Less Or Equal?(x=w269, y=w268) -> (x <= y?=w264:bool)
                n91 = Select(t="PASS", s=w264, f="FAIL") -> (s? t:f=w265:string)
              }
              frame Disabled {
              }
            }
            n92 = call "CSVFormat_Rx.vi"() -> ()  [unwired: 11 in, 1 out]
            n93 = call "CSVFormat_Rx.vi"("TV Parameters(DataType)"=w227, "WLAN RX Result"=w228) -> ("Rx Row"=w226:string[])  [unwired: 9 in]
            n94 = Current VI's Path() -> (path=w243:path)
            n95 = Strip Path(path=w243) -> (stripped path=w242:path)  [unwired: 1 out]
            n96 = Concatenate Strings(w236, "_Report.txt" ("string")) -> (w244:string)
            n97 = Build Path(base path=w242, name or relative path=w244) -> ()  [unwired: 1 out]
            n98 = Replace Array Subset(array=w235, new element=w233, index=9) -> ()  [unwired: 1 out]
            n99 = Number To Fractional String(number=w241, precision (6)=i16 3) -> (F-format string=w261:string)  [unwired: 2 in]
            n100 = Number To Decimal String(number=w256) -> (decimal integer string=w258:string)  [unwired: 1 in]
            n101 = Number To Fractional String(number=w240, precision (6)=i16 2) -> (F-format string=w249:string)  [unwired: 2 in]
            n102 = Number To Decimal String(number=w253) -> (decimal integer string=w255:string)  [unwired: 1 in]
            n103 = Concatenate Strings("Test Time = ", w261, " s" ("string"), w239) -> (w259:string)
            n104 = Concatenate Strings("GOOD_PACKETS : " ("string"), w258, w239) -> (w248:string)
            n105 = Concatenate Strings("PER : " ("string"), w249, " %" ("string"), w233, w239) -> (w246:string)
            n106 = Concatenate Strings("TOTAL_PACKETS : " ("string"), w255, w239) -> (w247:string)
            n107 = Equal?(x=w236, y=T9 "DUT 1") -> ()  [unwired: 1 out]
            n108 = Build Array(w259, w248, w247, w246) -> ()  [unwired: 1 out]
            n109 = call-poly <vilib>:"Write To Spreadsheet File.vi"("delimiter (\\t)"="," ("delimiter (\\t)"), "append to file? (new file:F)"=TRUE, "1D data"=w226, "file path (dialog if empty)"=w231) -> ("new file path (Not A Path if cancelled)"=w237:path)  [unwired: 4 in]
          }
          frame "Append Customized Text" {
            n110 = Current VI's Path() -> (path=w281:path)
            n111 = Strip Path(path=w281) -> (stripped path=w280:path)  [unwired: 1 out]
            n112 = Concatenate Strings(w276, "_Report.txt" ("string")) -> (w282:string)
            n113 = Build Array(w272) -> (w273:string[][])
            n114 = Build Path(base path=w280, name or relative path=w282) -> ()  [unwired: 1 out]
            n115 = Equal?(x=w276, y=T9 "DUT 1") -> ()  [unwired: 1 out]
            n116 = call-poly <vilib>:"Write To Spreadsheet File.vi"("delimiter (\\t)"="," ("delimiter (\\t)"), "append to file? (new file:F)"=TRUE, "1D data"=w272, "file path (dialog if empty)"=w278) -> ("new file path (Not A Path if cancelled)"=w277:path)  [unwired: 4 in]
          }
          frame "Read Log File" {
            n117 = Current VI's Path() -> (path=w294:path)
            n118 = Strip Path(path=w294) -> (stripped path=w293:path)  [unwired: 1 out]
            n119 = Concatenate Strings(w292, "_Report.txt" ("string")) -> (w295:string)
            n120 = Build Path(base path=w293, name or relative path=w295) -> ()  [unwired: 1 out]
            n121 = call-poly <vilib>:"Read From Spreadsheet File.vi"("delimiter (\\t)"="," ("delimiter (\\t)"), "file path (dialog if empty)"=w291) -> ("all rows"=w284:string[][])  [unwired: 5 in, 4 out]
            "DUT1 Results" <- w284
            n122 = call "Results search.vi"("Results"=w284) -> ("p/f"=w289:bool)  [unwired: 10 in]
            n123 = Bundle By Name(cluster=T10 {"all rows"=[], "p/f"=FALSE, "all rows"=[], "p/f"=FALSE} ("Cluster 2"), "all rows"=w284, "p/f"=w289, "all rows"=string[][] [], "p/f"=FALSE) -> (w287:T10)
          }
          frame "Save Test Time" {
            n124 = call "GetTime.vi"() -> ("TimeInSeconds"=w297:i32)  [unwired: 8 in, 3 out]
            n125 = Current VI's Path() -> (path=w304:path)
            n126 = Number To Fractional String(number=w297, precision (6)=i16 3) -> (F-format string=w308:string)  [unwired: 2 in]
            n127 = Strip Path(path=w304) -> (stripped path=w303:path)  [unwired: 1 out]
            n128 = Concatenate Strings(w302, "_Report.txt" ("string")) -> (w305:string)
            n129 = Concatenate Strings("------ Test Time = ", w308, " ------") -> (w300:string)
            n130 = Build Array(w300) -> (w299:string[])
            n131 = Build Path(base path=w303, name or relative path=w305) -> ()  [unwired: 1 out]
            n132 = call-poly <vilib>:"Write To Spreadsheet File.vi"("append to file? (new file:F)"=TRUE, "1D data"=w299, "file path (dialog if empty)"=w298) -> ()  [unwired: 5 in, 1 out]
          }
        }
      }
      "DUT1 log path" <- w20
      n133 = Compound Arithmetic op=AND(w26, w25, w24) -> (w23:bool)
    }
    frame Error {
    }
  }
  "error out" <- w11
  "Text Output" <- w9
  "Cluster 2" <- w8
  "Pass or not" <- w7
